vi "RSZVB Marker Target Search.vi"(7 "Search (0: Target Search)":i32(ring) items=["Target Search", "Target Search >", "< Target Search"], 8 "error in (no error)":errorcluster {"code" format="%.0x"}, 9 "Marker (1)":i32=1, 10 "Channel (Trace) (1)":i32=1, 11 "VISA session":refnum<visa-resource-name>) -> (0 "error out":errorcluster {"code" format="%.0x"}, 3 "dup VISA session":refnum<visa-resource-name>)   [LabVIEW 2011]
doc: "This VI search with the active marker for target value on the trace.\n\nNote(s):\n\nThe marker must be created before using CALCulate<Ch/Tr>:MARKer<Mk>[:STATe] ON.\n\nRemote-control command(s):\nCALCulate<Ch/Tr>:MARKer<Mk>:FUNCtion:EXECute TARGet | RTARget | LTARget"
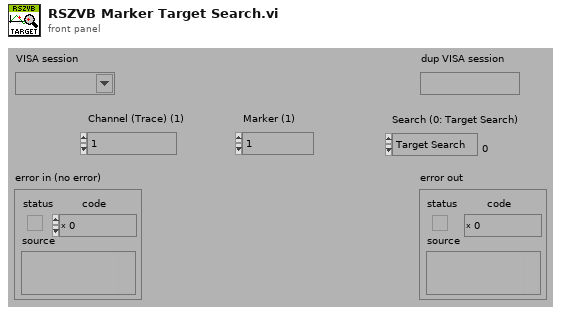
[diagram p1: front panel]
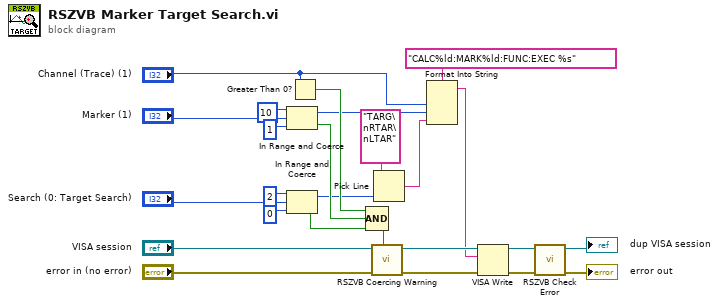
[diagram p0: block diagram]
diagram:
  n1 = In Range and Coerce(upper limit=10, x="Marker (1)", lower limit=1) -> (coerced(x)=w16:i32, In Range?=w17:bool)
  n2 = In Range and Coerce(upper limit=2, x="Search (0: Target Search)", lower limit=0) -> (coerced(x)=w12:i32, In Range?=w8:bool)
  n3 = Greater Than 0?(x="Channel (Trace) (1)") -> (x > 0?=w20:bool)
  n4 = Compound Arithmetic op=AND(w20, w17, w8) -> (w10:bool)
  n5 = call "RSZVB Coercing Warning.vi"("In Range?"=w10, "error in (no error)"="error in (no error)", "VISA session"="VISA session") -> ("error out"=w24:errorcluster, "dup VISA session"=w25:refnum<visa-resource-name>)  [unwired: 7 in]
  n6 = Pick Line(multi-line string="TARG\nRTAR\nLTAR", line index=w12) -> (output string=w11:string)  [unwired: 1 in]
  n7 = Format Into String(format string="CALC%ld:MARK%ld:FUNC:EXEC %s", "Channel (Trace) (1)", w16, w11) -> (resulting string=w9:string)  [unwired: 2 in, 1 out]
  n8 = VISA Write(VISA resource name=w25, write buffer=w9, error in (no error)=w24) -> (VISA resource name out=w22:refnum<visa-resource-name>, error out=w23:errorcluster)  [unwired: 1 out]
  n9 = call "RSZVB Check Error.vi"("error in (no error)"=w23, "VISA session"=w22) -> ("error out"=→"error out":errorcluster, "dup VISA session"=→"dup VISA session":refnum<visa-resource-name>)  [unwired: 8 in]
